vi "encodeObject.vi"(5 "Cluster To Map? (T)":bool=TRUE, 7 "Compress? (T)":bool=TRUE, 8 "error in (no error)":errorcluster, 11 "Variant":variant) -> (0 "error out":errorcluster, 3 "MessagePack":u8[](array[numeric]) format="%.0x")   [LabVIEW 2015, in "MsgPack.lvlib"]
uses:
  MsgPack.lvlib
  EncodeTypes/encodeInt8.vi
  EncodeTypes/encodeInt16.vi
  EncodeTypes/encodeInt32.vi
  EncodeTypes/encodeInt64.vi
  EncodeTypes/encodeUInt8.vi
  EncodeTypes/encodeUInt16.vi
  EncodeTypes/encodeUInt32.vi
  EncodeTypes/encodeUInt64.vi
  EncodeTypes/encodeFloat32.vi
  EncodeTypes/encodeFloat64.vi
  EncodeTypes/encodeString.vi
  EncodeTypes/encodeTimestamp.vi
  SubVis/encodeFixedInt.vi
  EncodeTypes/encodeExt.vi
  EncodeTypes/encodeBoolean.vi
  EncodeTypes/encodeArrayVariant.vi
  <vilib>/ErrorRing/Error Ring.xnode
  <vilib>/Utility/Data Type/NI_Data Type.lvlib
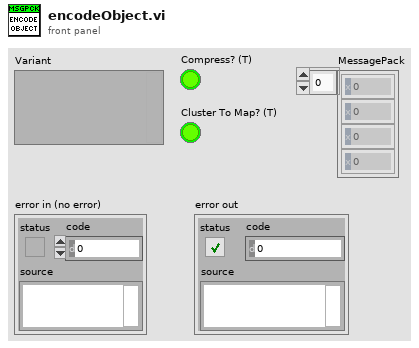
[diagram p1: front panel]
types:
  T1 = typedef "NI_Data Type.lvlib/Data Type.ctl" = enum8{"Invalid Type", "Void", "I8", "I16", "I32", "I64", "U8", "U16", "U32", "U64", "Single Float", "Double Float", "Extended Float", "Single Complex", "Double Complex", "Extended Complex", "Enum U8", "Enum U16", "Enum U32", "Enum U64", "Single Float With Unit", "Double Float With Unit", "Extended Float With Unit", "Single Complex with Unit", "Double Complex with Unit", "Extended Complex with Unit", "Boolean", "String", "Path", "Picture", "Tag", "Array", "Cluster", "Variant", "LV Variant", "Waveform", "Timestamp", "Digital Waveform", "Digital Data", "ExpressData", "Refnum", "External Data", "VI", "Poly VI", "LabVIEW Class Instance", "Fixed Point"}
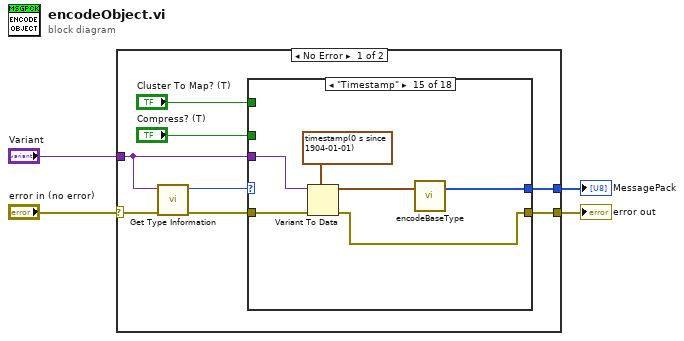
[diagram p0: block diagram]
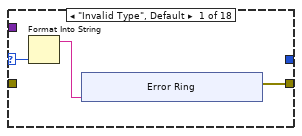
[diagram p2: hidden frame]
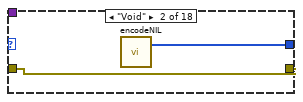
[diagram p3: hidden frame]
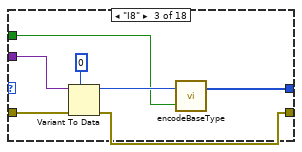
[diagram p4: hidden frame]
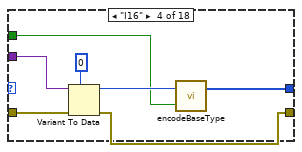
[diagram p5: hidden frame]
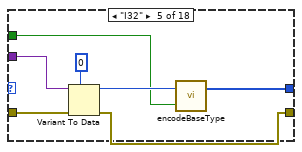
[diagram p6: hidden frame]
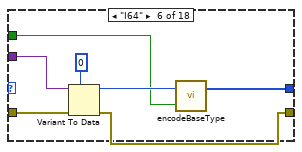
[diagram p7: hidden frame]
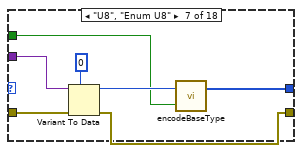
[diagram p8: hidden frame]
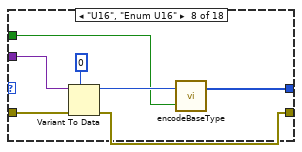
[diagram p9: hidden frame]
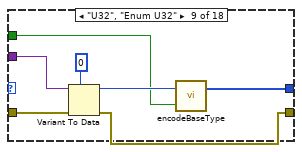
[diagram p10: hidden frame]
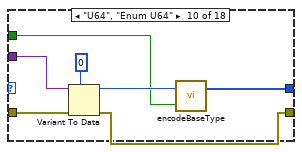
[diagram p11: hidden frame]
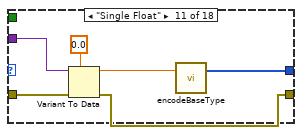
[diagram p12: hidden frame]
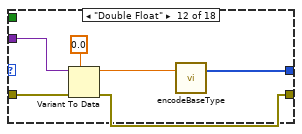
[diagram p13: hidden frame]
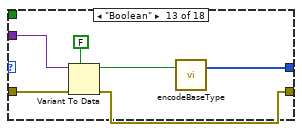
[diagram p14: hidden frame]
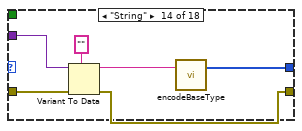
[diagram p15: hidden frame]
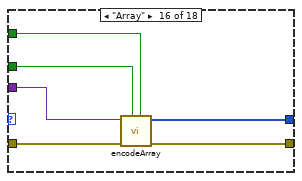
[diagram p16: hidden frame]
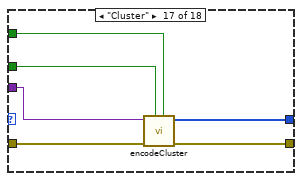
[diagram p17: hidden frame]
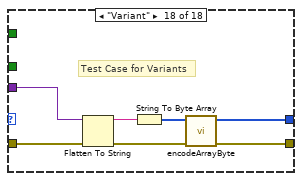
[diagram p18: hidden frame]
diagram:
  n1 = case shown="No Error" "error in (no error)" {
    selector: "error in (no error)" -> [w12 w128]
    tunnel: "Variant" -> [w11 _]
    tunnel: [w9 w128] -> w3
    tunnel: [w8 _] -> w2
    frame No Error {
      n2 = call <vilib>:"Get Type Information.vi"("error in (no error)"=w12, "Variant"=w11) -> ("error out"=w10:errorcluster, "Type"=w6:T1)  [unwired: 5 in, 3 out]
      n3 = case shown="\"Timestamp\"" w6 {
        selector: w6 -> [w14 _ _ _ _ _ _ _ _ _ _ _ _ _ _ _ _ _]
        tunnel: [w13 w22 w24 w31 w38 w45 w52 w59 w66 w73 w79 w85 w92 w98 w104 w114 w116 w121] -> w9
        tunnel: w10 -> [_ w22 w28 w35 w42 w49 w56 w63 w70 w77 w83 w89 w95 w101 w107 w113 w115 w125]
        tunnel: w11 -> [_ _ w29 w36 w43 w50 w57 w64 w71 w78 w84 w90 w96 w102 w108 w111 w120 w126]
        tunnel: [_ w21 w26 w33 w40 w47 w54 w61 w68 w75 w81 w87 w93 w99 w105 w112 w117 w127] -> w8
        tunnel: "Compress? (T)" -> [_ _ w23 w30 w37 w44 w51 w58 w65 w72 _ _ _ _ _ w110 w119 _]
        tunnel: "Cluster To Map? (T)" -> [_ _ _ _ _ _ _ _ _ _ _ _ _ _ _ w109 w118 _]
        frame "Invalid Type", Default {
          n4 = Format Into String(w14) -> (resulting string=w15:string)  [unwired: 3 in, 1 out]
          n5 = xnode "Error Ring"("parameter 0"=w15) -> ("error out"=w13:errorcluster)
        }
        frame "Void" {
          n6 = call "encodeNIL.vi"() -> ("MessagePack"=w21:u8[])  [unwired: 3 in]
        }
        frame "I8" {
          n7 = Variant To Data(error in=w28, type=i8 0, Variant=w29) -> (data=w27:i8, error out=w24:errorcluster)
          n8 = call-poly "encodeBaseType.vi"("Compress? (T)"=w23, "Int8"=w27) -> ("MessagePack"=w26:u8[])  [unwired: 1 in]
        }
        frame "I16" {
          n9 = Variant To Data(error in=w35, type=i16 0, Variant=w36) -> (data=w34:i16, error out=w31:errorcluster)
          n10 = call-poly "encodeBaseType.vi"("Compress? (T)"=w30, "Int16"=w34) -> ("MessagePack"=w33:u8[])  [unwired: 1 in]
        }
        frame "I32" {
          n11 = Variant To Data(error in=w42, type=0, Variant=w43) -> (data=w41:i32, error out=w38:errorcluster)
          n12 = call-poly "encodeBaseType.vi"("Compress? (T)"=w37, "Int32"=w41) -> ("MessagePack"=w40:u8[])  [unwired: 1 in]
        }
        frame "I64" {
          n13 = Variant To Data(error in=w49, type=i64 0, Variant=w50) -> (data=w48:i64, error out=w45:errorcluster)
          n14 = call-poly "encodeBaseType.vi"("Compress? (T)"=w44, "Int64"=w48) -> ("MessagePack"=w47:u8[])  [unwired: 1 in]
        }
        frame "U8", "Enum U8" {
          n15 = Variant To Data(error in=w56, type=u8 0, Variant=w57) -> (data=w55:u8, error out=w52:errorcluster)
          n16 = call-poly "encodeBaseType.vi"("Compress? (T)"=w51, "UInt8"=w55) -> ("MessagePack"=w54:u8[])  [unwired: 1 in]
        }
        frame "U16", "Enum U16" {
          n17 = Variant To Data(error in=w63, type=u16 0, Variant=w64) -> (data=w62:u16, error out=w59:errorcluster)
          n18 = call-poly "encodeBaseType.vi"("Compress? (T)"=w58, "UInt16"=w62) -> ("MessagePack"=w61:u8[])  [unwired: 1 in]
        }
        frame "U32", "Enum U32" {
          n19 = Variant To Data(error in=w70, type=u32 0, Variant=w71) -> (data=w69:u32, error out=w66:errorcluster)
          n20 = call-poly "encodeBaseType.vi"("Compress? (T)"=w65, "UInt32"=w69) -> ("MessagePack"=w68:u8[])  [unwired: 1 in]
        }
        frame "U64", "Enum U64" {
          n21 = Variant To Data(error in=w77, type=u64 0, Variant=w78) -> (data=w76:u64, error out=w73:errorcluster)
          n22 = call-poly "encodeBaseType.vi"("Compress? (T)"=w72, "UInt64"=w76) -> ("MessagePack"=w75:u8[])  [unwired: 1 in]
        }
        frame "Single Float" {
          n23 = Variant To Data(error in=w83, type=sgl 0.0, Variant=w84) -> (data=w82:sgl, error out=w79:errorcluster)
          n24 = call-poly "encodeBaseType.vi"("Float32"=w82) -> ("MessagePack"=w81:u8[])  [unwired: 2 in]
        }
        frame "Double Float" {
          n25 = Variant To Data(error in=w89, type=0.0, Variant=w90) -> (data=w88:dbl, error out=w85:errorcluster)
          n26 = call-poly "encodeBaseType.vi"("Float64"=w88) -> ("MessagePack"=w87:u8[])  [unwired: 2 in]
        }
        frame "Boolean" {
          n27 = Variant To Data(error in=w95, type=FALSE, Variant=w96) -> (data=w94:bool, error out=w92:errorcluster)
          n28 = call-poly "encodeBaseType.vi"("Boolean"=w94) -> ("MessagePack"=w93:u8[])  [unwired: 2 in]
        }
        frame "String" {
          n29 = Variant To Data(error in=w101, type="", Variant=w102) -> (data=w100:string, error out=w98:errorcluster)
          n30 = call-poly "encodeBaseType.vi"("string"=w100) -> ("MessagePack"=w99:u8[])  [unwired: 2 in]
        }
        frame "Timestamp" {
          n31 = Variant To Data(error in=w107, type=timestamp(0 s since 1904-01-01), Variant=w108) -> (data=w106:timestamp, error out=w104:errorcluster)
          n32 = call-poly "encodeBaseType.vi"("Time Stamp"=w106) -> ("MessagePack"=w105:u8[])  [unwired: 2 in]
        }
        frame "Array" {
          n33 = call-poly "encodeArray.vi"("Cluster To Map? (T)"=w109, "Compress? (T)"=w110, "error in"=w113, "Variant"=w111) -> ("error out"=w114:errorcluster, "MessagePack"=w112:u8[])  [unwired: 6 in]
        }
        frame "Cluster" {
          n34 = call "encodeCluster.vi"("Cluster To Map? [T]"=w118, "Compress? (T)"=w119, "error in (no error)"=w115, "Variant"=w120) -> ("error out"=w116:errorcluster, "MessagePack"=w117:u8[])  [unwired: 6 in]
        }
        frame "Variant" {
          # "Test Case for Variants"
          n35 = Flatten To String(anything=w126, error in (no error)=w125) -> (data string=w124:string, error out=w122:errorcluster)  [unwired: 2 in, 1 out]
          n36 = String To Byte Array(string=w124) -> (unsigned byte array=w123:u8[])
          n37 = call "encodeArrayByte.vi"("error in (no error)"=w122, "Byte Array"=w123) -> ("error out"=w121:errorcluster, "MessagePack"=w127:u8[])  [unwired: 8 in]
        }
      }
    }
    frame Error {
    }
  }
  "MessagePack" <- w2
  "error out" <- w3
